vi "Vision Processing For Cool People.vi"(3 "Range":cluster{"Lower value":sgl, "Upper value":sgl}={"Lower value"=234.67392, "Upper value"=255.0} {"Lower value" scale=0.0..255.0; "Upper value" scale=0.0..255.0}, 4 "Image Size":T2, 5 "View 2":bool, 6 "Original Image":T3(plugin-control)) -> (0 "Position":cluster{"X":dbl, "Y":dbl}, 1 "Processed Image":T3(plugin-control), 2 "Target Info":T1(array[cluster]))   [LabVIEW 2011]
uses:
  <vilib>/Rock Robotics/WPI/Camera/WPI_CameraImageSize.ctl
  <vilib>/vision/NI_Vision_Development_Module.lvlib
panel:
  in  "4":bool
  in  "3":bool
  in  "2":bool
  in  "1":bool
  in  "Processing":enum32{"Color", "Intensity", "Intensity Open"}(tab)=enum."Intensity"
  in  "Luminance":i32=255
  in  "Saturation":i32=255
  in  "Hue":i32(knob)=65 scale=0.0..255.0
  in  "Margins":cluster{"Hue":i32, "Sat":i32, "Lum":i32}={"Hue"=20, "Sat"=27, "Lum"=30} {"Sat" scale=0.0..40.0; "Lum" scale=0.0..40.0; "Hue" scale=0.0..40.0}
  in  "Range 2":cluster{"Lower value":sgl, "Upper value":sgl}={"Lower value"=234.67392, "Upper value"=255.0} {"Lower value" scale=0.0..255.0; "Upper value" scale=0.0..255.0}
  in  "Particle Count Limit":i32=8
  in  "Area Size Limit":i32=444
  in  "Score Limits":T4={"Rect Coverage"=76.0, "Aspect Ratio"=70.0, "X Edge Strength"=40.0, "Y Edge Strength"=60.0}
  in  "Camera Type":enum16{"206", "1011"}(ring)=enum."1011"
  in  "View":bool
  out "Original Image 2":T3(plugin-control)
  # "This SubVI gets a camera picture from the Dashboard, marks rectangular shapes and finds their\nDistance (in inches or meters).\nColor Processing finds the target by it's color. However, should the target be lighted with any sort of flashlight\npointing roughly at the same direction as the Camera's lens, it's easier to use Intensity Processing as the rectangular targets\nare Retro-Reflective and it's very easy to distinguish their intensity."
  # "Camera type affects:\n1. Extracting a single plane from a color image (useful for Intensity Processing) \n2. Camera's view angle for distance calculation."
  # "Note: the X and Y values are measured from the target's center.\nDistance is measured from the camera's lens to the target's center."
  # "That's the indicator of the original image."
  # "That's the control the SubVI receives as an input."
  # "That's the processed image."
  # "RECOMMENDED\nLower value: 234\nUpper value: 255\nConsidering the retro-reflective target is lighted"
  # "RECOMMENDED\nLower value: 234\nUpper value: 255\nConsidering the retro-reflective target is lighted"
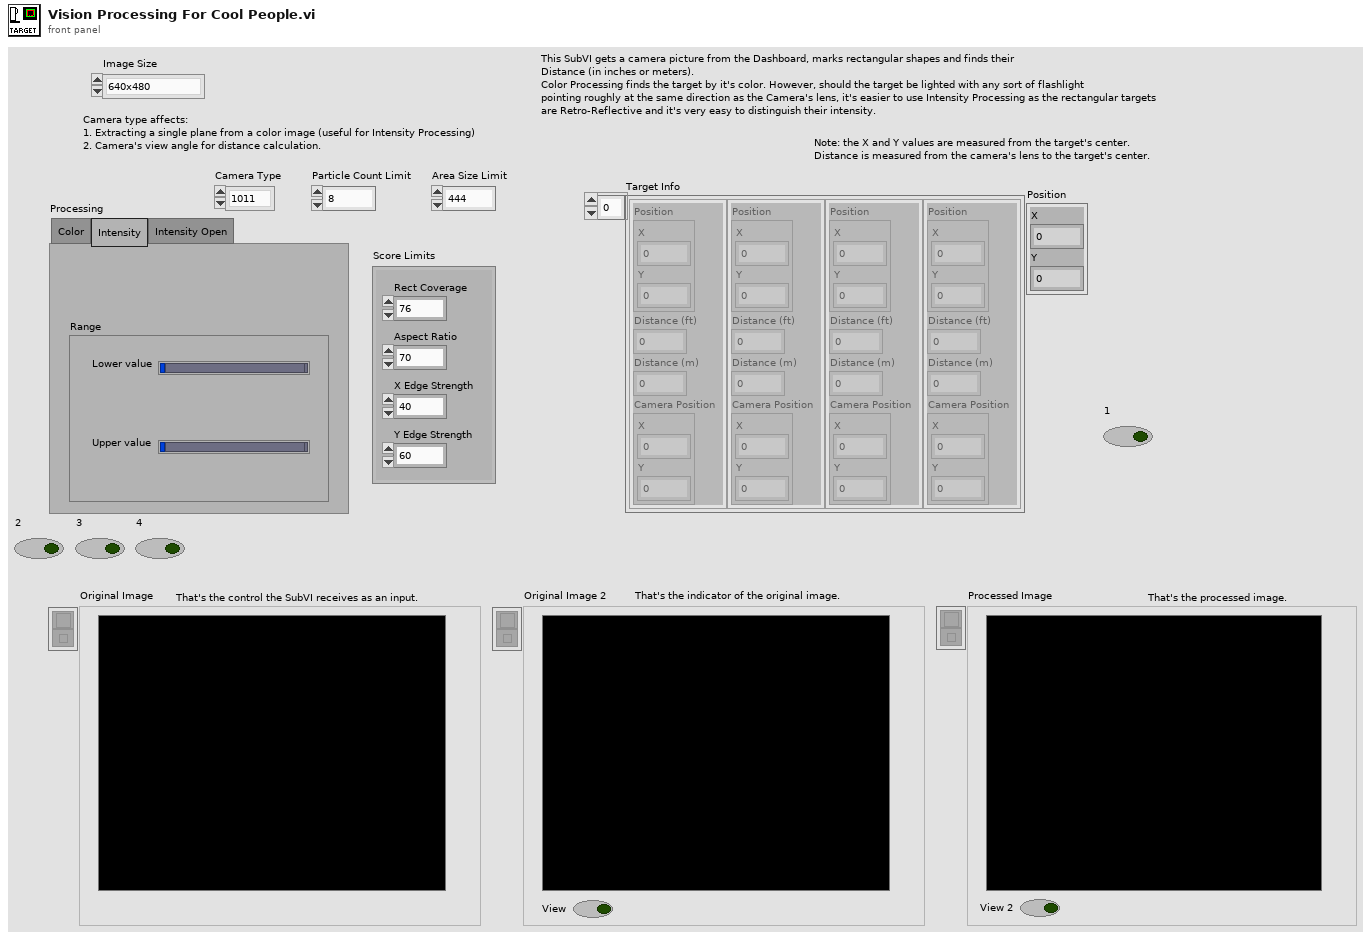
[diagram p1: front panel]
types:
  T1 = cluster{"Position":cluster{"X":dbl, "Y":dbl}, "Distance (ft)":dbl, "Distance (m)":dbl, "Camera Position":cluster{"X":dbl, "Y":dbl}}[]
  T2 = typedef "WPI_CameraImageSize.ctl" = enum16{"640x480", "320x240", "160x120"}
  T3 = typedef "IMAQ Image.ctl" = refnum<image>
  T4 = cluster{"Rect Coverage":dbl, "Aspect Ratio":dbl, "X Edge Strength":dbl, "Y Edge Strength":dbl}
  T5 = typedef "Image Type" = u32
  T6 = enum32{"AutoM", "Close", "Dilate", "Erode", "Gradient", "Gradient out", "Gradient in", "Hit miss", "Open", "PClose", "POpen", "Thick", "Thin"}
  T7 = cluster{cluster{"Left":dbl, "Top":dbl, "Right":dbl, "Bottom":dbl}, dbl[]}[]
  T8 = cluster{"Left":dbl, "Top":dbl, "Right":dbl, "Bottom":dbl}
  T9 = cluster{"Target Center (-1 to 1)":cluster{"X":dbl, "Y":dbl}, "Distance (ft)":dbl, "Distance (m)":dbl, "Target Center (Camera)":cluster{"X":dbl, "Y":dbl}}
  T10 = cluster{"Target Center (-1 to 1)":cluster{"X":dbl, "Y":dbl}, "Distance (ft)":dbl, "Distance (m)":dbl, "Target Center (Camera)":cluster{"X":dbl, "Y":dbl}}[]
  T11 = cluster{"Position":cluster{"X":dbl, "Y":dbl}, "Distance (ft)":dbl, "Distance (m)":dbl, "Camera Position":cluster{"X":dbl, "Y":dbl}}
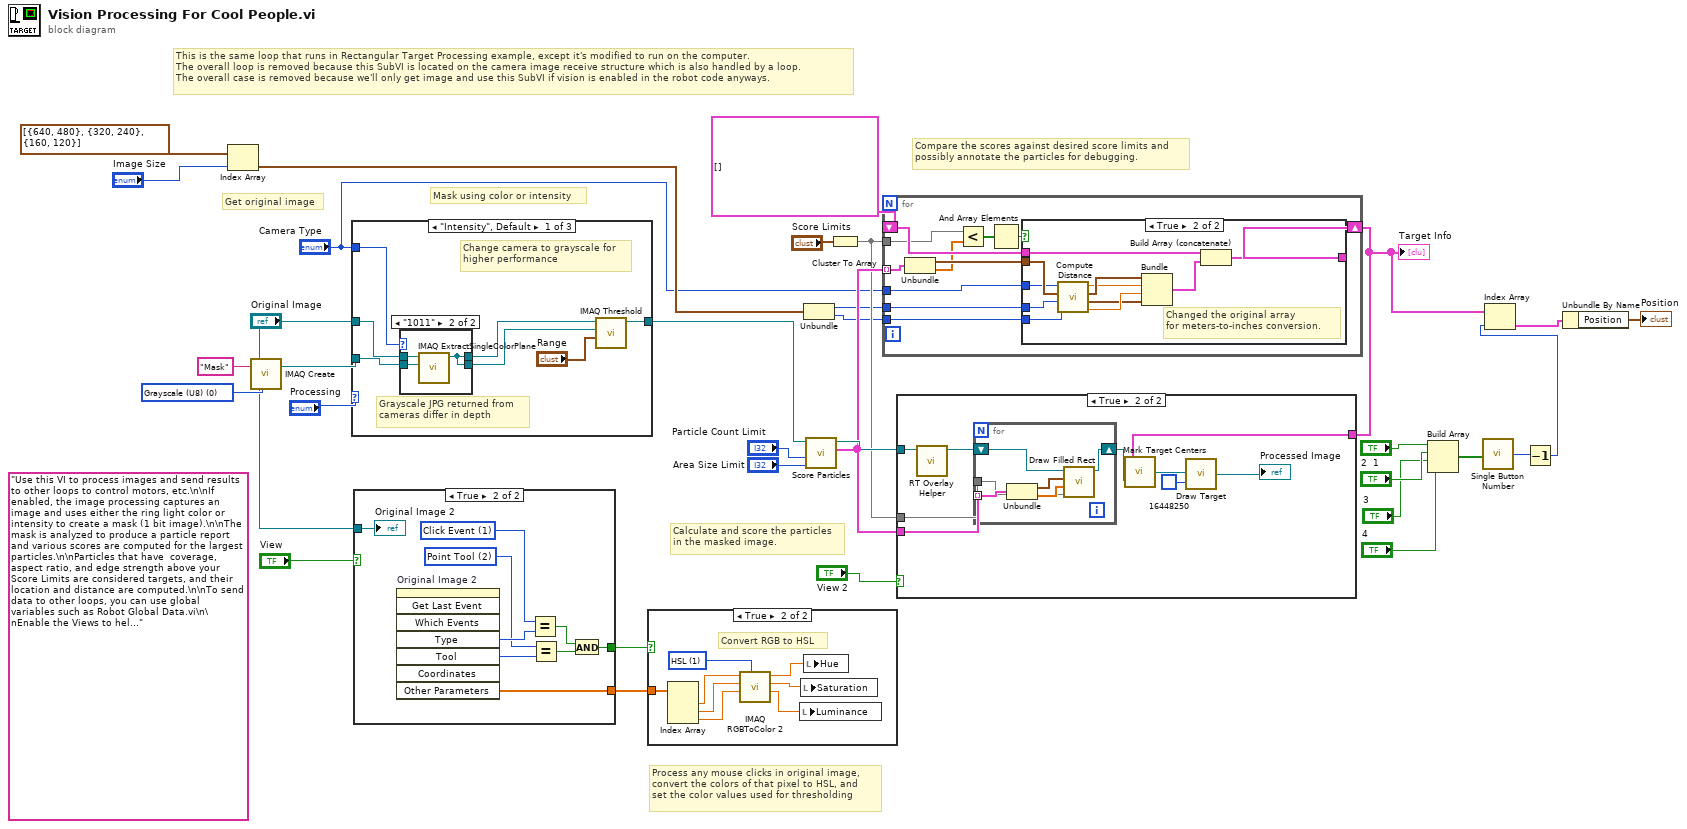
[diagram p0: block diagram]
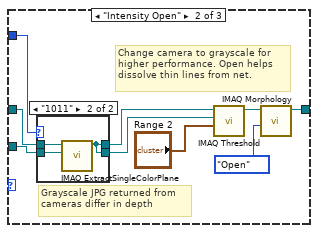
[diagram p4: hidden frame]
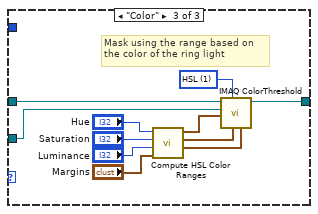
[diagram p6: hidden frame]
diagram:
  w33 = T5 0 items=["Grayscale (U8)", "Grayscale (I16)", "Grayscale (SGL)", "Complex (CSG)", "RGB (U32)", "HSL (U32)", "RGB (U64)", "Grayscale (U16)"] ("Image Type")
  (unwired) "Use this VI to process images and send results to other loops to control motors, etc.\n\nIf enabled, the image processing captures an image and uses either the ring light color or intensity to create a mask (1 bit image).\n\nThe mask is analyzed to produce a particle report and various scores are computed for the largest particles.\n\nParticles that have  coverage, aspect ratio, and edge strength above your Score Limits are considered targets, and their location and distance are computed.\n\nTo send data to other loops, you can use global variables such as Robot Global Data.vi\n\nEnable the Views to help debug color settings. Disable the View to speed up processing."
  # "Compare the scores against desired score limits and\npossibly annotate the particles for debugging."
  # "Process any mouse clicks in original image,\nconvert the colors of that pixel to HSL, and\nset the color values used for thresholding"
  # "Calculate and score the particles\nin the masked image."
  # "Mask using color or intensity"
  # "Get original image"
  # "This is the same loop that runs in Rectangular Target Processing example, except it's modified to run on the computer.\nThe overall loop is removed because this SubVI is located on the camera image receive structure which is also handled by a loop.\nThe overall case is removed because we'll only get image and use this SubVI if vision is enabled in the robot code anyways."
  n1 = Index Array(array=cluster{i32, i32}[] [{640, 480}, {320, 240}, {160, 120}], index="Image Size") -> (element=w13:cluster{i32, i32})
  n2 = call "IMAQ Create"("Image Name"="Mask", "Image Type"=w33) -> ("New Image"=w31:T3)  [unwired: 2 in, 2 out]
  n3 = case shown="\"Intensity\", Default" "Processing" {
    tunnel: "Original Image" -> [w38 w48 w70]
    tunnel: [w39 w51 w69] -> w18
    tunnel: w31 -> [w37 w49 w60]
    tunnel: "Camera Type" -> [w36 w50 _]
    frame "Intensity", Default {
      # "Grayscale JPG returned from\ncameras differ in depth"
      # "Change camera to grayscale for\nhigher performance"
      n4 = case shown="\"1011\"" w36 {
        tunnel: w38 -> [w42 w45]
        tunnel: w37 -> [w41 w44]
        tunnel: [w42 w43] -> w35
        tunnel: [w41 w43] -> w34
        frame "206", Default {
        }
        frame "1011" {
          n5 = call "IMAQ ExtractSingleColorPlane"("Image Dst"=w44, "Image Src"=w45) -> ("Image Dst Out"=w43:T3)  [unwired: 8 in, 1 out]
        }
      }
      n6 = call "IMAQ Threshold"("Range"="Range", "Image Dst"=w34, "Image Src"=w35) -> ("Image Dst Out"=w39:T3)  [unwired: 3 in, 5 out]
    }
    frame "Intensity Open" {
      # "Grayscale JPG returned from\ncameras differ in depth"
      # "Change camera to grayscale for\nhigher performance. Open helps\ndissolve thin lines from net."
      n7 = case shown="\"1011\"" w50 {
        tunnel: w48 -> [w56 w59]
        tunnel: w49 -> [w55 w58]
        tunnel: [w56 w57] -> w47
        tunnel: [w55 w57] -> w46
        frame "206", Default {
        }
        frame "1011" {
          n8 = call "IMAQ ExtractSingleColorPlane"("Image Dst"=w58, "Image Src"=w59) -> ("Image Dst Out"=w57:T3)  [unwired: 8 in, 1 out]
        }
      }
      n9 = call "IMAQ Threshold"("Range"="Range 2", "Image Dst"=w46, "Image Src"=w47) -> ("Image Dst Out"=w52:T3)  [unwired: 3 in, 5 out]
      n10 = call "IMAQ Morphology"("Operation"=T6."Open", "Image Src"=w52) -> ("Image Dst Out"=w51:T3)  [unwired: 8 in, 1 out]
    }
    frame "Color" {
      w68 = u16 1 items=["RGB", "HSL", "HSV", "HSI"] ("Color Mode")
      # "Mask using the range based on\nthe color of the ring light"
      n11 = call "Compute HSL Color Ranges.vi"("Margins"="Margins", "Luminance"="Luminance", "Saturation"="Saturation", "Hue"="Hue") -> ("Lum Range"=w65:cluster{i32, i32}, "Sat Range"=w66:cluster{i32, i32}, "Hue Range"=w67:cluster{i32, i32})  [unwired: 5 in]
      n12 = call "IMAQ ColorThreshold"("Blue or Luma or Val or Inten Range"=w65, "Green or Sat Range"=w66, "Color Mode"=w68, "Red or Hue Range"=w67, "Image Dst"=w60, "Image Src"=w70) -> ("Image Dst Out"=w69:T3)  [unwired: 4 in, 1 out]
    }
  }
  n13 = case shown="True" "View" {
    tunnel: "Original Image" -> [_ w79]
    tunnel: [_ w74] -> w17
    tunnel: [_ w71] -> w16
    frame False {
    }
    frame True {
      w72 = 2 items=["None", "Selection Tool", "Point Tool", "Line Tool", "Rectangle Tool", "Oval Tool", "Polygon Tool", "ClosedFreehandTool", "Annulus Tool", "Rotated Rectangle Tool", "Zoom Tool", "Pan Tool", "Polyline Tool", "Freehand Tool"] ("Tool")
      w73 = 1 items=["No Event"=0, "Click Event"=1, "Draw Event"=2, "Size Event"=4, "Scroll Event"=5, "Double Click Event"=8] ("Type")
      n14 = invoke on="Original Image 2" class="ImageControl" method="Get Last Event"() -> ("Type"=w75:i32, "Tool"=w78:i32, "Other Parameters"=w71:sgl[])  [unwired: 8 in, 5 out]
      n15 = Equal?(x=w73, y=w75) -> (x = y?=w76:bool)
      n16 = Equal?(x=w72, y=w78) -> (x = y?=w77:bool)
      n17 = And(x=w76, y=w77) -> (x .and. y?=w74:bool)
      "Original Image 2" <- w79
    }
  }
  n18 = case shown="True" w17 {
    tunnel: w16 -> [_ w87]
    frame False {
    }
    frame True {
      w86 = u16 1 items=["RGB", "HSL", "HSV", "HSI", "CIE L*a*b*", "CIE XYZ"] ("Color Mode")
      # "Convert RGB to HSL"
      n19 = Index Array(array=w87) -> (element #1=w85:sgl, element #2=w83:sgl, element #3=w81:sgl)  [unwired: 3 in]
      n20 = call "IMAQ RGBToColor 2"("Color Mode"=w86, "Blue value"=w81, "Green value"=w83, "Red value"=w85) -> ("Blue or Luma or Val or Inten or Z or b*value"=w80:dbl, "Green or Sat or Y or a* value"=w82:dbl, "Red or Hue or X or L* value"=w84:dbl)  [unwired: 4 in, 1 out]
      n21 = local write "Luminance"(w80) -> ()
      n22 = local write "Saturation"(w82) -> ()
      n23 = local write "Hue"(w84) -> ()
    }
  }
  n24 = Unbundle(w13) -> (w15:i32, w14:i32)
  n25 = call "Score Particles.vi"("Area Size Limit"="Area Size Limit", "Particle Count Limit"="Particle Count Limit", "Image Refnum in"=w18) -> ("Scored Particle Info"=w24:T7, "Image Refnum out"=w27:T3)  [unwired: 7 in]
  n26 = Cluster To Array(cluster="Score Limits") -> (array=w22:dbl[])
  n27 = for {
    shift-right: [w97] -> w4
    shift-left: T1 [] -> [w98]
    tunnel: w15 -> [w96]
    tunnel: w24 -> [w94] mode=indexing
    tunnel: w22 -> [w89]
    tunnel: "Camera Type" -> [w93]
    tunnel: w14 -> [w88]
    n28 = Unbundle(w94) -> (w95:T8, w90:dbl[])
    n29 = Less?(x=w89, y=w90) -> (x < y?=w92:bool[])
    n30 = And Array Elements(Boolean array=w92) -> (logical AND=w91:bool)
    n31 = case shown="True" w91 {
      tunnel: w98 -> [w99 w110]
      tunnel: [w99 w100] -> w97
      tunnel: w95 -> [_ w108]
      tunnel: w96 -> [_ w109]
      tunnel: w93 -> [_ w107]
      tunnel: w88 -> [_ w106]
      frame False {
      }
      frame True {
        # "Changed the original array\nfor meters-to-inches conversion."
        n32 = call "Compute Distance.vi"("Y Image Resolution"=w106, "X Image Resolution"=w109, "Bounding Box"=w108, "Camera Type"=w107) -> ("Distance (m)"=w102:dbl, "Target Center (Camera)"=w101:cluster{"X":dbl, "Y":dbl}, "Target Center (-1 to 1)"=w104:cluster{"X":dbl, "Y":dbl}, "Distance (ft)"=w103:dbl)  [unwired: 4 in]
        n33 = Bundle("Target Center (-1 to 1)"=w104, "Distance (ft)"=w103, "Distance (m)"=w102, "Target Center (Camera)"=w101) -> (w105:T9)  [unwired: 1 in]
        n34 = Build Array (concatenate)(w110, w105) -> (w100:T10)
      }
    }
  }
  "Target Info" <- w4
  n35 = case shown="True" "View 2" {
    tunnel: w27 -> [_ w116]
    tunnel: w24 -> [_ w118]
    tunnel: w22 -> [_ w117]
    tunnel: w4 -> [_ w114]
    frame False {
    }
    frame True {
      n36 = call "RT Overlay Helper.vi"("Refnum in"=w116) -> ("Refnum out"=w119:T3)  [unwired: 10 in]
      n37 = for {
        shift-right: [w124] -> w115
        shift-left: w119 -> [w125]
        tunnel: w118 -> [w121] mode=indexing
        tunnel: w117 -> [w120]
        n38 = Unbundle(w121) -> (w122:T8, w123:dbl[])
        n39 = call "Draw Filled Rect.vi"("Limits"=w120, "Scores"=w123, "Bounding Box"=w122, "image in"=w125) -> ("image out"=w124:T3)  [unwired: 7 in]
      }
      n40 = call "Mark Target Centers.vi"("Processed Image"=w115, "Target Info"=w114) -> ("Image Out"=w113:T3)
      n41 = call "Draw Target.vi"("Color"=u32 16448250, "Original Image"=w113) -> ("Image Out"=→"Processed Image":T3)
    }
  }
  n42 = Build Array("1", "2", "3", "4") -> (w6:bool[])
  n43 = call "Single Button Number.vi"("Bool Array"=w6) -> ("Number"=w5:i32)
  n44 = Decrement(x=w5) -> (x-1=w3:i32)
  n45 = Index Array(array=w4, index=w3) -> (element=w2:T11)
  n46 = Unbundle By Name(w2) -> ("Position"=→"Position":cluster{"X":dbl, "Y":dbl})
